vi "main.vi"() -> ()   [LabVIEW 2016]
uses:
  INPUTS.ctl
  <vilib>/DAQmx/read.llb/DAQmx Read (Analog 2D DBL NChan NSamp).vi
  <vilib>/DAQmx/configure/timing.llb/DAQmx Timing (Sample Clock).vi
  <vilib>/DAQmx/miscellaneous.llb/DAQmx Fill In Error Info.vi
panel:
  out "I_CELL":dbl format="%0.2f"
  out "I_LOAD":dbl format="%0.2f"
  out "I_PV":dbl format="%0.2f"
  out "V_CELL":dbl format="%0.2f"
  out "V_BUS":dbl format="%0.2f"
  out "Currents":cluster{dbl[], dbl[]}[](graph) caption="VCC"
  out "Voltages":cluster{dbl[], dbl[]}[](graph) caption="VCC"
  in  "stop":bool
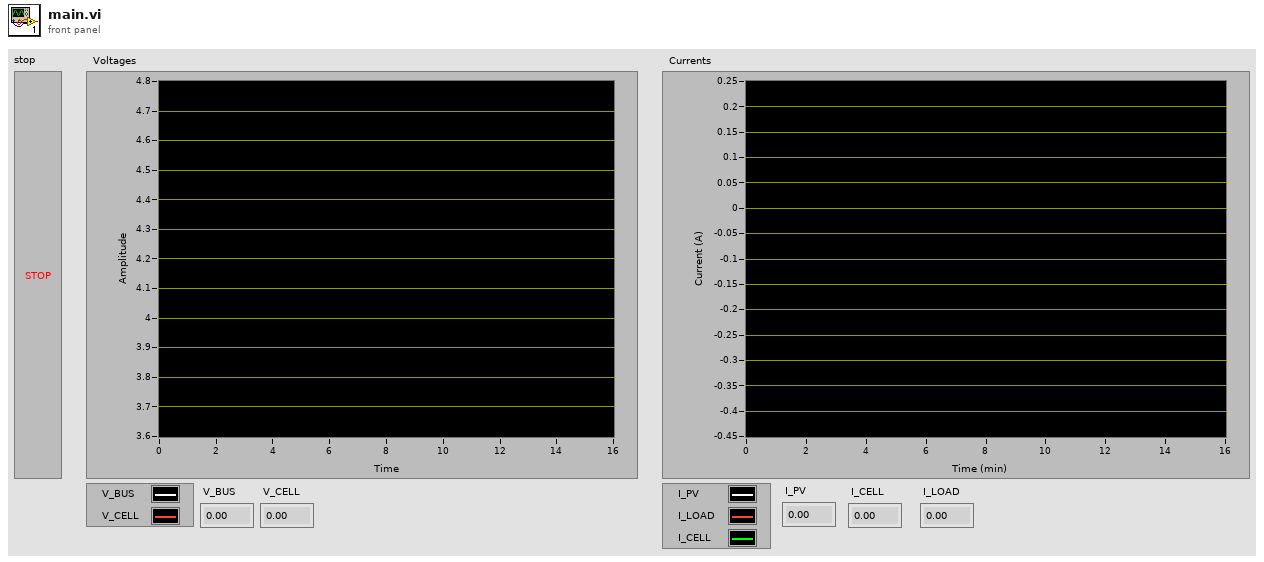
[diagram p1: front panel]
types:
  T1 = enum16{"open", "open or create", "create or replace", "create", "open (read only)"}
  T2 = typedef "INPUTS.ctl" = enum16{"VCC", "I_PV", "I_LOAD", "I_CELL", "V_BUS", "V_CELL"}
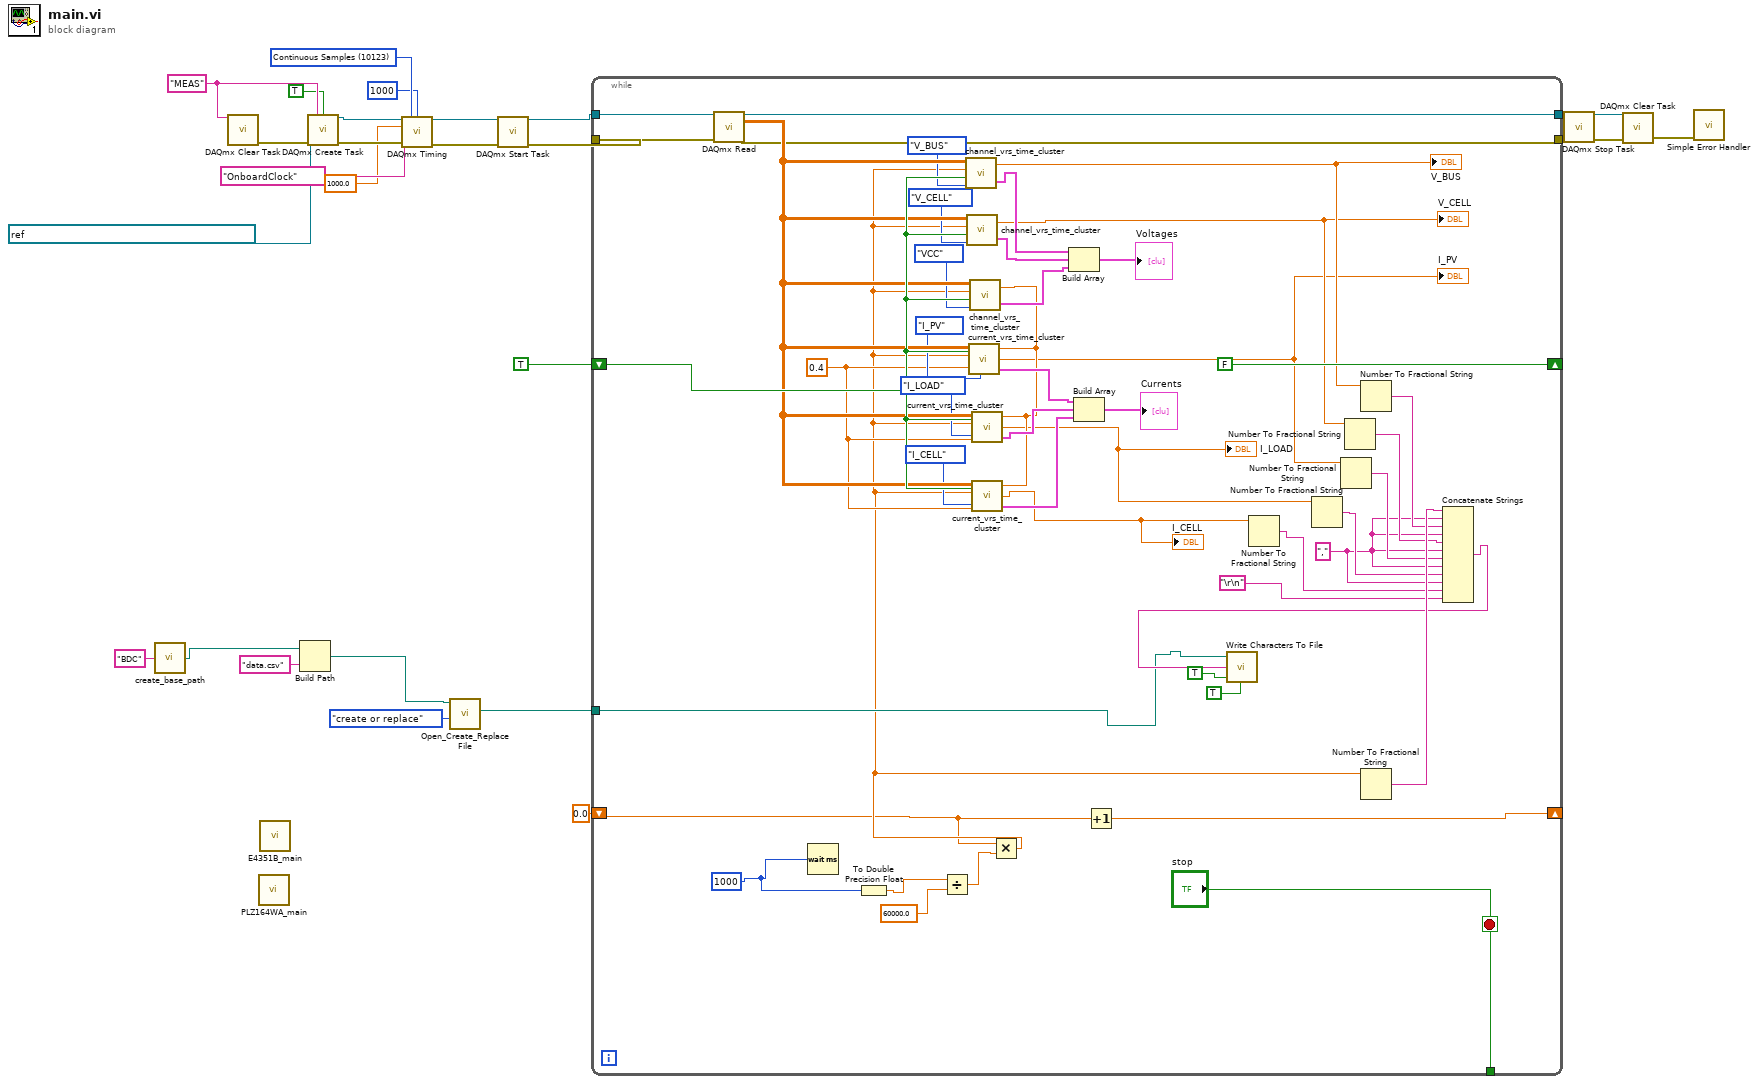
[diagram p0: block diagram]
diagram:
  w22 = 10123 items=["Finite Samples"=10178, "Continuous Samples"=10123, "Hardware Timed Single Point"=12522] ("sample mode")
  w9 = "MEAS" ("new task name")
  n1 = call "create_base_path.vi"("project name"="BDC") -> ("base path"=w3:path)
  n2 = call <vilib>:"DAQmx Clear Task.vi"("task in"=w9) -> ("error out"=w10:errorcluster)  [unwired: 14 in]
  n3 = call "PLZ164WA_main.vi"() -> ()  [unwired: 12 in]
  n4 = call "E4351B_main.vi"() -> ()  [unwired: 1 in]
  n5 = Build Path(base path=w3, name or relative path="data.csv") -> (appended path=w5:path)
  n6 = call <vilib>:"DAQmx Create Task.vi"("new task name"=w9, "auto cleanup"=TRUE, "global virtual channels"=refnum<k21> "VCC, I_PV, I_LOAD, I_CELL, V_BUS, V_CELL", "error in"=w10) -> ("task out"=w24:refnum<k21>, "error out"=w23:errorcluster)  [unwired: 10 in]
  n7 = call-poly <vilib>:"DAQmx Timing.vi"("task/channels in"=w24, "sample mode"=w22, "samples per channel"=1000, "rate"=1000.0, "source"=tag "OnboardClock", "error in"=w23) -> ("task out"=w19:refnum<k21>, "error out"=w18:errorcluster)  [unwired: 8 in]
  n8 = call <vilib>:"Open_Create_Replace File.vi"("function (open:0)"=T1."create or replace", "file path"=w5) -> ("new file path"=w1:path)  [unwired: 6 in, 3 out]
  n9 = call <vilib>:"DAQmx Start Task.vi"("task/channels in"=w19, "error in"=w18) -> ("task out"=w17:refnum<k21>, "error out"=w16:errorcluster)  [unwired: 12 in]
  n10 = while {
    shift-right: [w28] -> _
    shift-left: 0.0 -> [w29]
    shift-right: [FALSE ("Clear Graph?")] -> _
    shift-left: TRUE ("Clear Graph?") -> [w68]
    tunnel: w17 -> [w70]
    tunnel: w16 -> [w69]
    tunnel: [w66] -> w15
    tunnel: [w65] -> w14
    tunnel: w1 -> [w32]
    tunnel: ["stop"] -> _
    stop <- "stop" stop-if-true
    w35 = "," ("string")
    w50 = 0.4 ("sensitivity (V/A)")
    w71 = u32 1000 ("milliseconds to wait")
    n11 = call-poly <vilib>:"DAQmx Read.vi"("task/channels in"=w70, "error in"=w69) -> ("task out"=w66:refnum<k21>, "data"=w67:dbl[][], "error out"=w65:errorcluster)  [unwired: 11 in]
    n12 = Wait (ms)(milliseconds to wait=w71) -> ()  [unwired: 1 out]
    n13 = To Double Precision Float(number=w71) -> (double precision float=w74:dbl)
    n14 = Divide(x=w74, y=60000.0) -> (x/y=w72:dbl)
    n15 = Multiply(x=w29, y=w72) -> (x*y=w31:dbl)
    n16 = call "channel_vrs_time_cluster.vi"("Enum"=INPUTS."V_BUS", "Clear Graph?"=w68, "Time"=w31, "Input data"=w67) -> ("Cluster"=w62:cluster{dbl[], dbl[]}, "rms value"=w45:dbl)
    "V_BUS" <- w45
    n17 = call "channel_vrs_time_cluster.vi"("Enum"=INPUTS."V_CELL", "Clear Graph?"=w68, "Time"=w31, "Input data"=w67) -> ("Cluster"=w61:cluster{dbl[], dbl[]}, "rms value"=w44:dbl)
    "V_CELL" <- w44
    n18 = call "channel_vrs_time_cluster.vi"("Enum"=INPUTS."VCC", "Clear Graph?"=w68, "Time"=w31, "Input data"=w67) -> ("Cluster"=w59:cluster{dbl[], dbl[]}, "rms value"=w49:dbl)
    n19 = call "current_vrs_time_cluster.vi"("Input data"=w67, "Clear Graph?"=w68, "Time"=w31, "Enum"=INPUTS."I_PV", "sensitivity (V/A)"=w50, "VCC"=w49) -> ("rms value"=w43:dbl, "Cluster"=w53:cluster{dbl[], dbl[]})  [unwired: 1 in]
    "I_PV" <- w43
    n20 = call "current_vrs_time_cluster.vi"("Input data"=w67, "Clear Graph?"=w68, "Time"=w31, "Enum"=INPUTS."I_LOAD", "sensitivity (V/A)"=w50, "VCC"=w49) -> ("rms value"=w42:dbl, "Cluster"=w52:cluster{dbl[], dbl[]})  [unwired: 1 in]
    "I_LOAD" <- w42
    n21 = call "current_vrs_time_cluster.vi"("Input data"=w67, "Clear Graph?"=w68, "Time"=w31, "Enum"=INPUTS."I_CELL", "sensitivity (V/A)"=w50, "VCC"=w49) -> ("rms value"=w41:dbl, "Cluster"=w51:cluster{dbl[], dbl[]})  [unwired: 1 in]
    "I_CELL" <- w41
    n22 = Build Array(w62, w61, w59) -> (→"Voltages":cluster{dbl[], dbl[]}[])
    n23 = Build Array(w53, w52, w51) -> (→"Currents":cluster{dbl[], dbl[]}[])
    n24 = Increment(x=w29) -> (x+1=w28:dbl)
    n25 = Number To Fractional String(number=w41) -> (F-format string=w34:string)  [unwired: 3 in]
    n26 = Number To Fractional String(number=w42) -> (F-format string=w36:string)  [unwired: 3 in]
    n27 = Number To Fractional String(number=w43) -> (F-format string=w37:string)  [unwired: 3 in]
    n28 = Number To Fractional String(number=w44) -> (F-format string=w38:string)  [unwired: 3 in]
    n29 = Number To Fractional String(number=w45) -> (F-format string=w39:string)  [unwired: 3 in]
    n30 = Number To Fractional String(number=w31) -> (F-format string=w46:string)  [unwired: 3 in]
    n31 = Concatenate Strings(w46, w35, w39, w35, w38, w35, w37, w35, w36, w35, w34, "\r\n") -> (w40:string)
    n32 = call <vilib>:"Write Characters To File.vi"("convert eol? (no:F)"=TRUE, "append to file? (new file:F)"=TRUE, "character string"=w40, "file path (dialog if empty)"=w32) -> ()  [unwired: 1 in, 1 out]
  }
  n33 = call <vilib>:"DAQmx Stop Task.vi"("task/channels in"=w15, "error in"=w14) -> ("task out"=w13:refnum<k21>, "error out"=w12:errorcluster)  [unwired: 12 in]
  n34 = call <vilib>:"DAQmx Clear Task.vi"("task in"=w13, "error in"=w12) -> ("error out"=w11:errorcluster)  [unwired: 13 in]
  n35 = call <vilib>:"Simple Error Handler.vi"("error in (no error)"=w11) -> ()  [unwired: 4 in, 5 out]
